vi "Example 5 (Get FPGA Scalars).vi"() -> ()   [LabVIEW 2018]
uses:
  <vilib>/addons/VeriStand Custom Device Scripting APIs/FPGA Addon/Scripting API.lvlibp/APIs/Scripting API/TypeDefs/Output Scalar Data.ctl
  <vilib>/addons/VeriStand Custom Device Scripting APIs/FPGA Addon/Scripting API.lvlibp/Addon/Addon Shared/Types/Data Type.ctl
  <vilib>/addons/VeriStand Custom Device Scripting APIs/FPGA Addon/Scripting API.lvlibp
  <vilib>/addons/VeriStand Custom Device Scripting APIs/FPGA Addon/Scripting API.lvlibp/Addon/Addon Shared/FPGA Addon Shared.lvlib
panel:
  out "size(s)":i32
  out "bitfile scalars out":T1[](array[typedef])
  out "error out":errorcluster
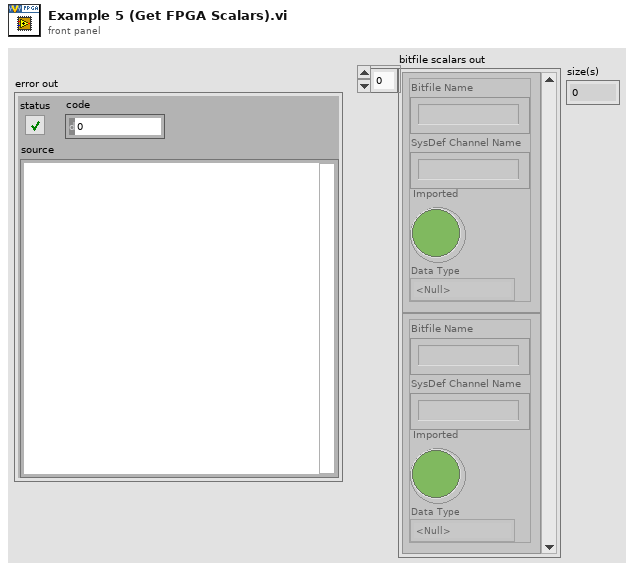
[diagram p1: front panel]
types:
  T1 = typedef "Scripting API.lvlibp/Output Scalar Data.ctl" = cluster{"Bitfile Name":string, "SysDef Channel Name":string, "Imported":bool, "Data Type":T2}
  T2 = typedef "Scripting API.lvlibp/FPGA Addon Shared.lvlib/Data Type.ctl" = enum8{"<Null>", "I8", "I16", "I32", "I64", "U8", "U16", "U32", "U64", "SGL", "Boolean", "Analog PWM In Settings", "Analog PWM In", "Digital PWM In Settings", "Digital PWM In", "Digital PWM Out", "Sine Out", "FXP+/-24.5", "FXP+/-16.5", "FXP+/-32.8", "FXP+/-64.32", "FXP+/-16.7", "FXP+/-20.5", "FXP+/-27.5", "FXP+/-32.16", "FXP+16.3", "FXP+18.3", "Digital Static In", "Digital Static Out", "Digital Static In Settings", "Digital WSS Out", "Quad Encoder Settings", "Quad Encoder In", "Group"}
  T3 = typedef "Scripting API.lvlibp/Custom Device API.lvlib/Custom Device Item Ref.ctl" = u64
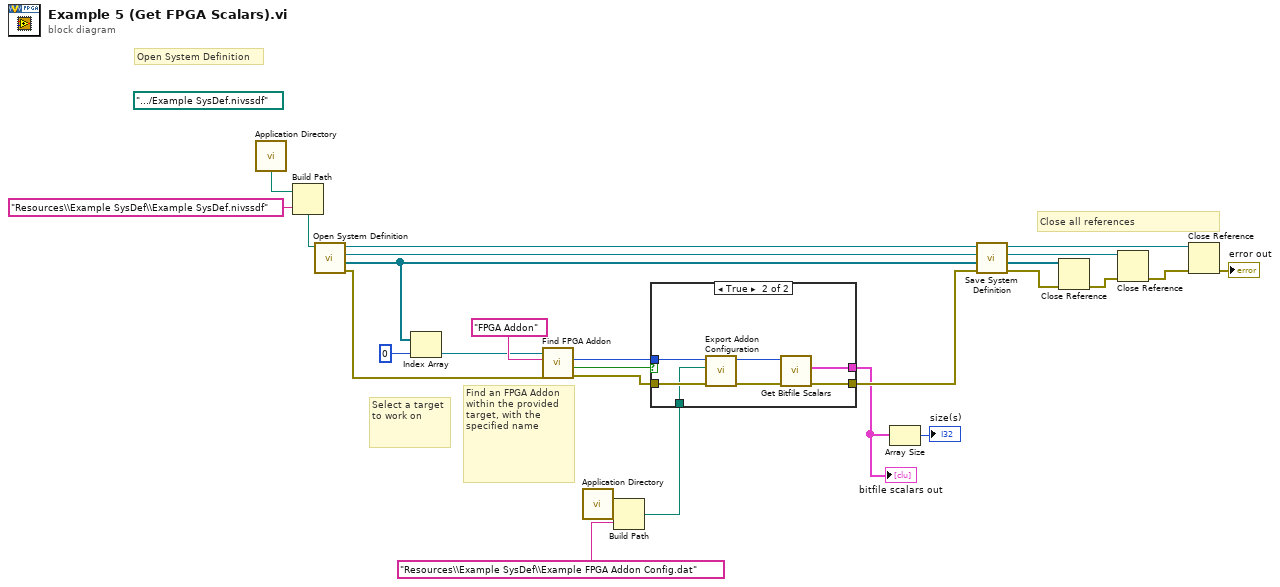
[diagram p0: block diagram]
diagram:
  (unwired) path ".../Example SysDef.nivssdf" ("fpga bitfile path")
  # "Close all references"
  # "Find an FPGA Addon within the provided target, with the specified name"
  # "Select a target to work on"
  # "Open System Definition"
  n1 = call <vilib>:"Application Directory.vi"() -> ("Application Directory"=w19:path)
  n2 = Build Path(base path=w19, name or relative path="Resources\\Example SysDef\\Example SysDef.nivssdf") -> (appended path=w17:path)
  n3 = call "Open System Definition.vi"("System Definition File"=w17) -> ("error out"=w3:errorcluster, "targets refnums"=w22:refnum<k24>[], "root refnum"=w23:refnum<k24>, "system definition refnum"=w15:refnum<k24>)  [unwired: 7 in]
  n4 = Index Array(array=w22, index=0) -> (element=w4:refnum<k24>)
  n5 = call <vilib>:"Find FPGA Addon.vi"("error in (no error)"=w3, "FPGA Addon name"="FPGA Addon" ("fpga addon name"), "target in"=w4) -> ("error out"=w10:errorcluster, "found ?"=w5:bool, "FPGA Addon refnum out"=w11:T3)  [unwired: 5 in, 1 out]
  n6 = call <vilib>:"Application Directory.vi"() -> ("Application Directory"=w9:path)
  n7 = Build Path(base path=w9, name or relative path="Resources\\Example SysDef\\Example FPGA Addon Config.dat") -> (appended path=w7:path)
  n8 = case shown="True" w5 {
    tunnel: w11 -> [_ w32]
    tunnel: w10 -> [w25 w31]
    tunnel: w7 -> [_ w30]
    tunnel: [w25 w27] -> w6
    tunnel: [_ w26] -> w2
    frame False {
    }
    frame True {
      n9 = call <vilib>:"Export Addon Configuration.vi"("error in (no error)"=w31, "export file path"=w30, "FPGA Addon refnum in"=w32) -> ("error out"=w29:errorcluster, "FPGA Addon refnum out"=w28:T3)  [unwired: 7 in]
      n10 = call <vilib>:"Get Bitfile Scalars.vi"("error in (no error)"=w29, "FPGA Addon refnum in"=w28) -> ("error out"=w27:errorcluster, "bitfile scalars out"=w26:T1[])  [unwired: 7 in, 1 out]
    }
  }
  "bitfile scalars out" <- w2
  n11 = Array Size(array=w2) -> (size(s)=→"size(s)":i32)
  n12 = call "Save System Definition.vi"("error in (no error)"=w6, ".NET Refnum in"=w15) -> ("error out"=w13:errorcluster, ".NET Refnum out"=w14:refnum<k24>)  [unwired: 8 in]
  n13 = Close Reference(reference=w22, error in (no error)=w13) -> (error out=w21:errorcluster)
  n14 = Close Reference(reference=w23, error in (no error)=w21) -> (error out=w20:errorcluster)
  n15 = Close Reference(reference=w14, error in (no error)=w20) -> (error out=→"error out":errorcluster)
